vi "Send OVP.vi"(8 "error in":errorcluster, 11 "6700C in":refnum<class "6700C.lvclass">) -> (0 "error out":errorcluster, 3 "6700C out":refnum<class "6700C.lvclass">)   [LabVIEW 2019, in "6700C.lvlib" / "6700C.lvclass"]
uses:
  Library/6700C.lvclass
  C:/Users/Public/Documents/Development/builds/Instruments/PowerSupply.lvlibp/Library/PowerSupply.lvclass
  Library/6700C.lvclass/6700C.ctl
  Accessors/Read Local Resource.vi
  Accessors/Write Local Resource.vi
  builds/Instruments/PowerSupply.lvlibp/Accessors/Read Active Channel.vi
  <instrlib>/Agilent N6700 Series/Agilent N6700 Series.lvlib
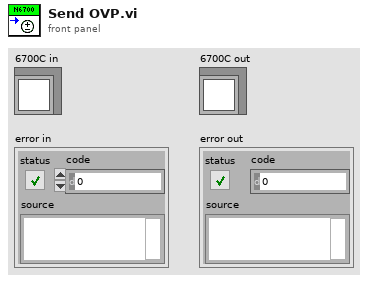
[diagram p1: front panel]
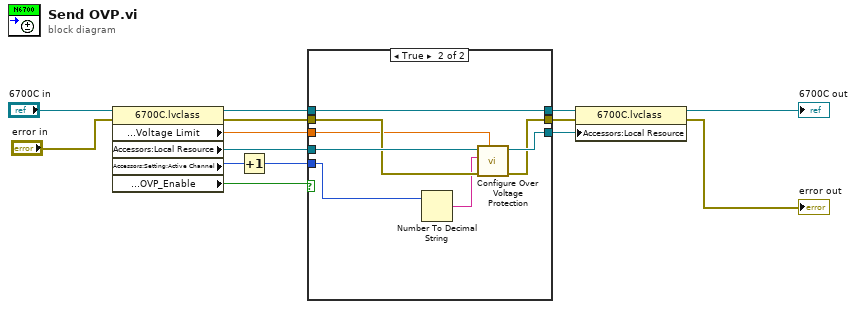
[diagram p0: block diagram]
diagram:
  n1 = property class="6700C.lvclass"(reference="6700C in", error in="error in") -> (reference out=w9:refnum<class "6700C.lvclass">, error out=w12:errorcluster, "Accessors:Setting:Protection:Voltage Limit"=w14:dbl, "Accessors:Local Resource"=w5:refnum<visa-resource-name>, "Accessors:Setting:Active Channel"=w4:u32, "Accessors:Setting:Protection:OVP_Enable"=w11:bool)
  n2 = Increment(x=w4) -> (x+1=w1:u32)
  n3 = case shown="True" w11 {
    tunnel: w1 -> [_ w19]
    tunnel: w5 -> [w15 w25]
    tunnel: [w15 w24] -> w6
    tunnel: w9 -> [w17 w23]
    tunnel: [w17 w23] -> w10
    tunnel: w12 -> [w16 w22]
    tunnel: [w16 w21] -> w13
    tunnel: w14 -> [_ w20]
    frame False {
    }
    frame True {
      n4 = Number To Decimal String(number=w19) -> (decimal integer string=w18:string)  [unwired: 1 in]
      n5 = call <instrlib>:"Configure Over Voltage Protection.vi"("Limit (0.0 volts)"=w20, "error in (no error)"=w22, "Channel Name (1)"=w18, "VISA resource name"=w25) -> ("error out"=w21:errorcluster, "VISA resource name out"=w24:refnum<visa-resource-name>)  [unwired: 6 in]
    }
  }
  n6 = property class="6700C.lvclass"(reference=w10, error in=w13, "Accessors:Local Resource"=w6) -> (reference out=→"6700C out":refnum<class "6700C.lvclass">, error out=→"error out":errorcluster)
